vi "waitTimeView.vi"(10 "UserEvents in":refnum<class "UserEvents.lvclass">) -> ()   [LabVIEW 2013, in "AITDTViews.lvlib"]
uses:
  AITDTViews.lvlib
  UserEvents/UserEvents.lvclass
  Typedefs/WaitTimeStatus.ctl
  UserEvents/UserEvents.lvclass/UserEvents.ctl
  Typedefs/StateSelector.ctl
  Typedefs/AITDTTypedefs.lvlib
panel:
  out "Wait Time Status":T1 {"Time Remaining" min=1.0 format="%.1f"}
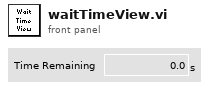
[diagram p1: front panel]
types:
  T1 = typedef "AITDTTypedefs.lvlib/WaitTimeStatus.ctl" = cluster{"Time Remaining":dbl[unit]}
  T2 = typedef "AITDTTypedefs.lvlib/PubDataEvents.ctl" = cluster{"State":refnum<user-event>, "ErrorCode":refnum<user-event>, "OutputData":refnum<user-event>, "InputData":refnum<user-event>, "TestStatus":refnum<user-event>, "LogPath":refnum<user-event>, "TemperatureSetpointRequest":refnum<user-event>, "TemperatureSettling":refnum<user-event>, "WaitTimeStatus":refnum<user-event>}
  T3 = cluster{"Event Registration Refnum":refnum<event-registration>, "Event Registration Refnum":refnum<event-registration>}
  T4 = typedef "AITDTTypedefs.lvlib/StateSelector.ctl" = enum16{"AwaitingSetpointAcknowledgmentState", "EndingCycleState", "FaultState", "OffState", "PausingState", "RequestingNewSetpointState", "SamplingState", "SettlingState", "SoakingState", "StabilizingState", "StandbyState", "StoppedState", "TransitioningTemperatureState"}
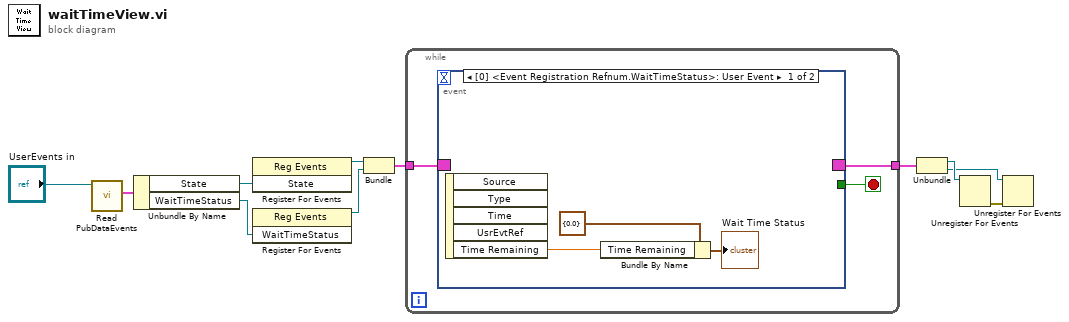
[diagram p0: block diagram]
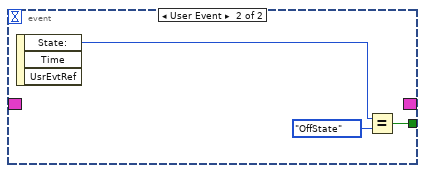
[diagram p2: hidden frame]
diagram:
  n1 = call "Read PubDataEvents.vi"("UserEvents in"="UserEvents in") -> ("PubDataEvents"=w11:T2)  [unwired: 9 in, 1 out]
  n2 = Unbundle By Name(w11) -> ("State"=w10:refnum<user-event>, "WaitTimeStatus"=w8:refnum<user-event>)
  n3 = register-events(w10) -> (reference out=w9:refnum<event-registration>)  [unwired: 2 in, 1 out]
  n4 = register-events(w8) -> (reference out=w7:refnum<event-registration>)  [unwired: 2 in, 1 out]
  n5 = Bundle("Event Registration Refnum"=w9, "Event Registration Refnum"=w7) -> (w5:T3)  [unwired: 1 in]
  n6 = while {
    tunnel: w5 -> [w14]
    tunnel: [w12] -> w4
    stop <- w13 stop-if-true
    n7 = event shown="[0] <Event Registration Refnum.WaitTimeStatus>: User Event" {
      selector: w14 -> [_ _]
      dyn-events: [_ _] -> w12
      timeout: _ -> [_ _]
      tunnel: [_ w19] -> w13
      event User Event {
        n8 = event-data() -> ("Time Remaining"=w16:dbl[unit])  [unwired: 1 in, 4 out]
        n9 = Bundle By Name(cluster=T1 {"Time Remaining"=0.0} ("Wait Time Status"), "Time Remaining"=w16) -> (→"Wait Time Status":T1)
      }
      event User Event {
        n10 = event-data() -> ("State:"=w18:T4)  [unwired: 1 in, 2 out]
        n11 = Equal?(x=w18, y=StateSelector."OffState" ("State:")) -> (x = y?=w19:bool)
      }
    }
  }
  n12 = Unbundle(w4) -> ("Event Registration Refnum"=w3:refnum<event-registration>, "Event Registration Refnum"=w2:refnum<event-registration>)
  n13 = Unregister For Events(event registration refnum=w3) -> (error out=w1:errorcluster)  [unwired: 1 in]
  n14 = Unregister For Events(event registration refnum=w2, error in=w1) -> ()  [unwired: 1 out]
